vi "Check.vi"(6 "Actions In":refnum<class "Iteration Actions.lvclass">, 7 "Report Conditions":bool, 9 "Sequence Time":T1, 10 "Variables":refnum<class "Variables.lvclass">, 11 "Transition in":refnum<class "Transition.lvclass">) -> (1 "Triggered":bool, 2 "Met Conditions":refnum<class "Condition.lvclass">[](array[class]), 3 "Transition out":refnum<class "Transition.lvclass">, 4 "Actions":refnum<class "Iteration Actions.lvclass">)   [LabVIEW 2020, in "VolatusSeq.lvlib" / "Transition.lvclass"]
uses:
  Transition.lvclass
  Iteration Actions/Iteration Actions.lvclass
  Variables/Variables.lvclass
  Sequence Time.ctl
  Condition/Condition.lvclass
  Transition.lvclass/Transition.ctl
  VolatusSeq.lvlib
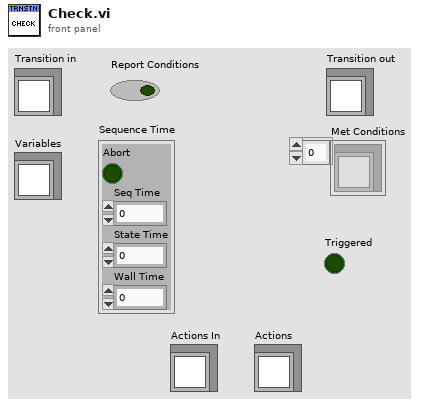
[diagram p1: front panel]
types:
  T1 = typedef "VolatusSeq.lvlib/Sequence Time.ctl" = cluster{"Abort":bool, "Seq Time":dbl, "State Time":dbl, "Wall Time":dbl}
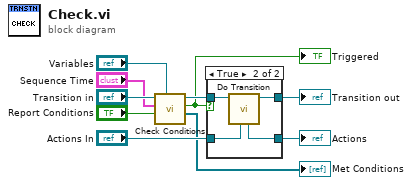
[diagram p0: block diagram]
diagram:
  n1 = call "Check Conditions.vi"("Variables"="Variables", "Report Conditions"="Report Conditions", "Sequence Time"="Sequence Time", "Transition in"="Transition in") -> ("Met Conditions"=→"Met Conditions":refnum<class "Condition.lvclass">[], "Met"=w5:bool, "Transition out"=w6:refnum<class "Transition.lvclass">)  [unwired: 5 in]
  "Triggered" <- w5
  n2 = case shown="True" w5 {
    tunnel: [w12 w16] -> w10
    tunnel: "Actions In" -> [w11 w15]
    tunnel: [w11 w14] -> w8
    tunnel: w6 -> [w12 w13]
    frame False {
    }
    frame True {
      n3 = call-dynamic "Do Transition.vi"("Actions In"=w15, "Transition in"=w13) -> ("Transition out"=w16:refnum<class "Transition.lvclass">, "Actions"=w14:refnum<class "Iteration Actions.lvclass">)  [unwired: 8 in]
    }
  }
  "Transition out" <- w10
  "Actions" <- w8
